vi "MultRRTPlan.vi"(6 "AttackerAvoidArea":bool=TRUE, 7 "Parameters.lvclass":refnum<class "Parameters.lvclass">, 8 "Volta ao redor\nda área?":bool, 9 "Line?":bool, 10 "IA State":T11={"our_robots"=[], "enemy_robots"=[], "balls"=[], "geometry"={"line_width"=0, "field_length"=0, "field_width"=0, "boundary_width"=0, "referee_width"=0, "goal_width"=0, "goal_depth"=0, "goal_wall_width"=0, "center_circle_radius"=0, "defense_radius"=0, "defense_stretch"=0, "free_kick_from_defense_dist"=0, "penalty_spot_from_field_line_dist"=0, "penalty_line_from_spot_dist"=0}, "IA Judge"={"stage"="", "command"="", "our_goalie_id"=0.0, "enemy_goalie_id"=0.0, "command enum"=enum."Halt", "Time"=enum."Azul", "Point"={"x"=0.0, "y"=0.0}}, "Received Timestamp"=timestamp(0 s since 1904-01-01), "Events"={"Touch"=FALSE, "Ball out"=FALSE, "id touch"=0.0, "Ball out of \nVision"=FALSE, "Ball inside \nGoalie area"=FALSE, "Robot not responding"=FALSE, "Robots responding status"=[1.0, 1.0, 1.0, 1.0, 1.0, 1.0], "Enemy Ball \nPossession"=FALSE, "Pass State"=FALSE, "id end of pass"=0.0, "Kick"=FALSE, "Id ini Possession"=0.0, "Ball Possesion"=FALSE, "Id Possesion"=0.0, "Direct Kick"=FALSE, "2nd Strk Ativo"=FALSE}}, 11 "Robot":T1={"id"=0, "function"=enum."Attacker", "x"=0.0, "y"=0.0, "orientation"=0.0, "v_tangent"=0.0, "v_normal"=0.0, "v_ang"=0.0, "kick_x"=0.0, "kick_z"=0.0, "dribble"=FALSE, "Timestamp"=timestamp(0 s since 1904-01-01), "estimatives"={"est_v_tangent"=0.0, "est_v_normal"=0.0, "est_vx"=0.0, "est_vy"=0.0, "Pos Robot Est"=[], "est_v_ang"=0.0}, "dest_x_kick"=0.0, "dest_y_kick"=0.0, "Gap Coord"=[], "States"=enum."GoToTangent", "Path "=[], "Path  Smooth"=[], "Dest"=[], "vx_desired"=0.0, "vy_desired"=0.0, "slowBehavior"=FALSE, "VSSStates"=enum."Pass", "robotKickState"=enum."none", "role"=enum."DefenderArea", "x_k|k"=[]}) -> (2 "Robot Out":T1={"id"=0, "function"=enum."Attacker", "x"=0.0, "y"=0.0, "orientation"=0.0, "v_tangent"=0.0, "v_normal"=0.0, "v_ang"=0.0, "kick_x"=0.0, "kick_z"=0.0, "dribble"=FALSE, "Timestamp"=timestamp(0 s since 1904-01-01), "estimatives"={"est_v_tangent"=0.0, "est_v_normal"=0.0, "est_vx"=0.0, "est_vy"=0.0, "Pos Robot Est"=[], "est_v_ang"=0.0}, "dest_x_kick"=0.0, "dest_y_kick"=0.0, "Gap Coord"=[], "States"=enum."GoToTangent", "Path "=[], "Path  Smooth"=[], "Dest"=[], "vx_desired"=0.0, "vy_desired"=0.0, "slowBehavior"=FALSE, "VSSStates"=enum."Pass", "robotKickState"=enum."none", "role"=enum."DefenderArea", "x_k|k"=[]})   [LabVIEW 2021]
uses:
  Vision_class/Old vision/Controls/AI Robot.ctl
  Vision_class/Old vision/Controls/Functions Enum.ctl
  Controls/estimatives.ctl
  Vision_class/Old vision/Controls/AttackerStates.ctl
  Vision_class/Old vision/Controls/PathDests.ctl
  Vision_class/Old vision/Controls/PathDest.ctl
  Navigation/VSSNavigation/VSSAttackerStates.ctl
  Robot_class/robotKickToStates.ctl
  Robot_class/roles.ctl
  <vilib>/Analysis/Matrix/Datatypes/RealMatrix.ctl
  Vision_class/Old vision/SSL Detection Frame Simple Estimator Cameras VelCmd Folder/Core/AI Input.ctl
  Vision_class/Old vision/SSL Detection Frame Simple Estimator Cameras VelCmd Folder/Core/AI Ball.ctl
  Vision_class/Old vision/SSL Detection Frame Simple Estimator Cameras VelCmd Folder/Core/Field Size.ctl
  Vision_class/Old vision/SSL Detection Frame Simple Estimator Cameras VelCmd Folder/Core/AI Judge.ctl
  Communication_class/Paths/MessageAI_State Folder/Intel/Command Enum.ctl
  Vision_class/Old vision/SSL Detection Frame Simple Estimator Cameras VelCmd Folder/Util/Events/Events.ctl
  Parameters_class/Parameters.lvclass
  Utilities_class/Utilities.lvclass
  <vilib>/Analysis/Matrix/NI_Matrix.lvlib
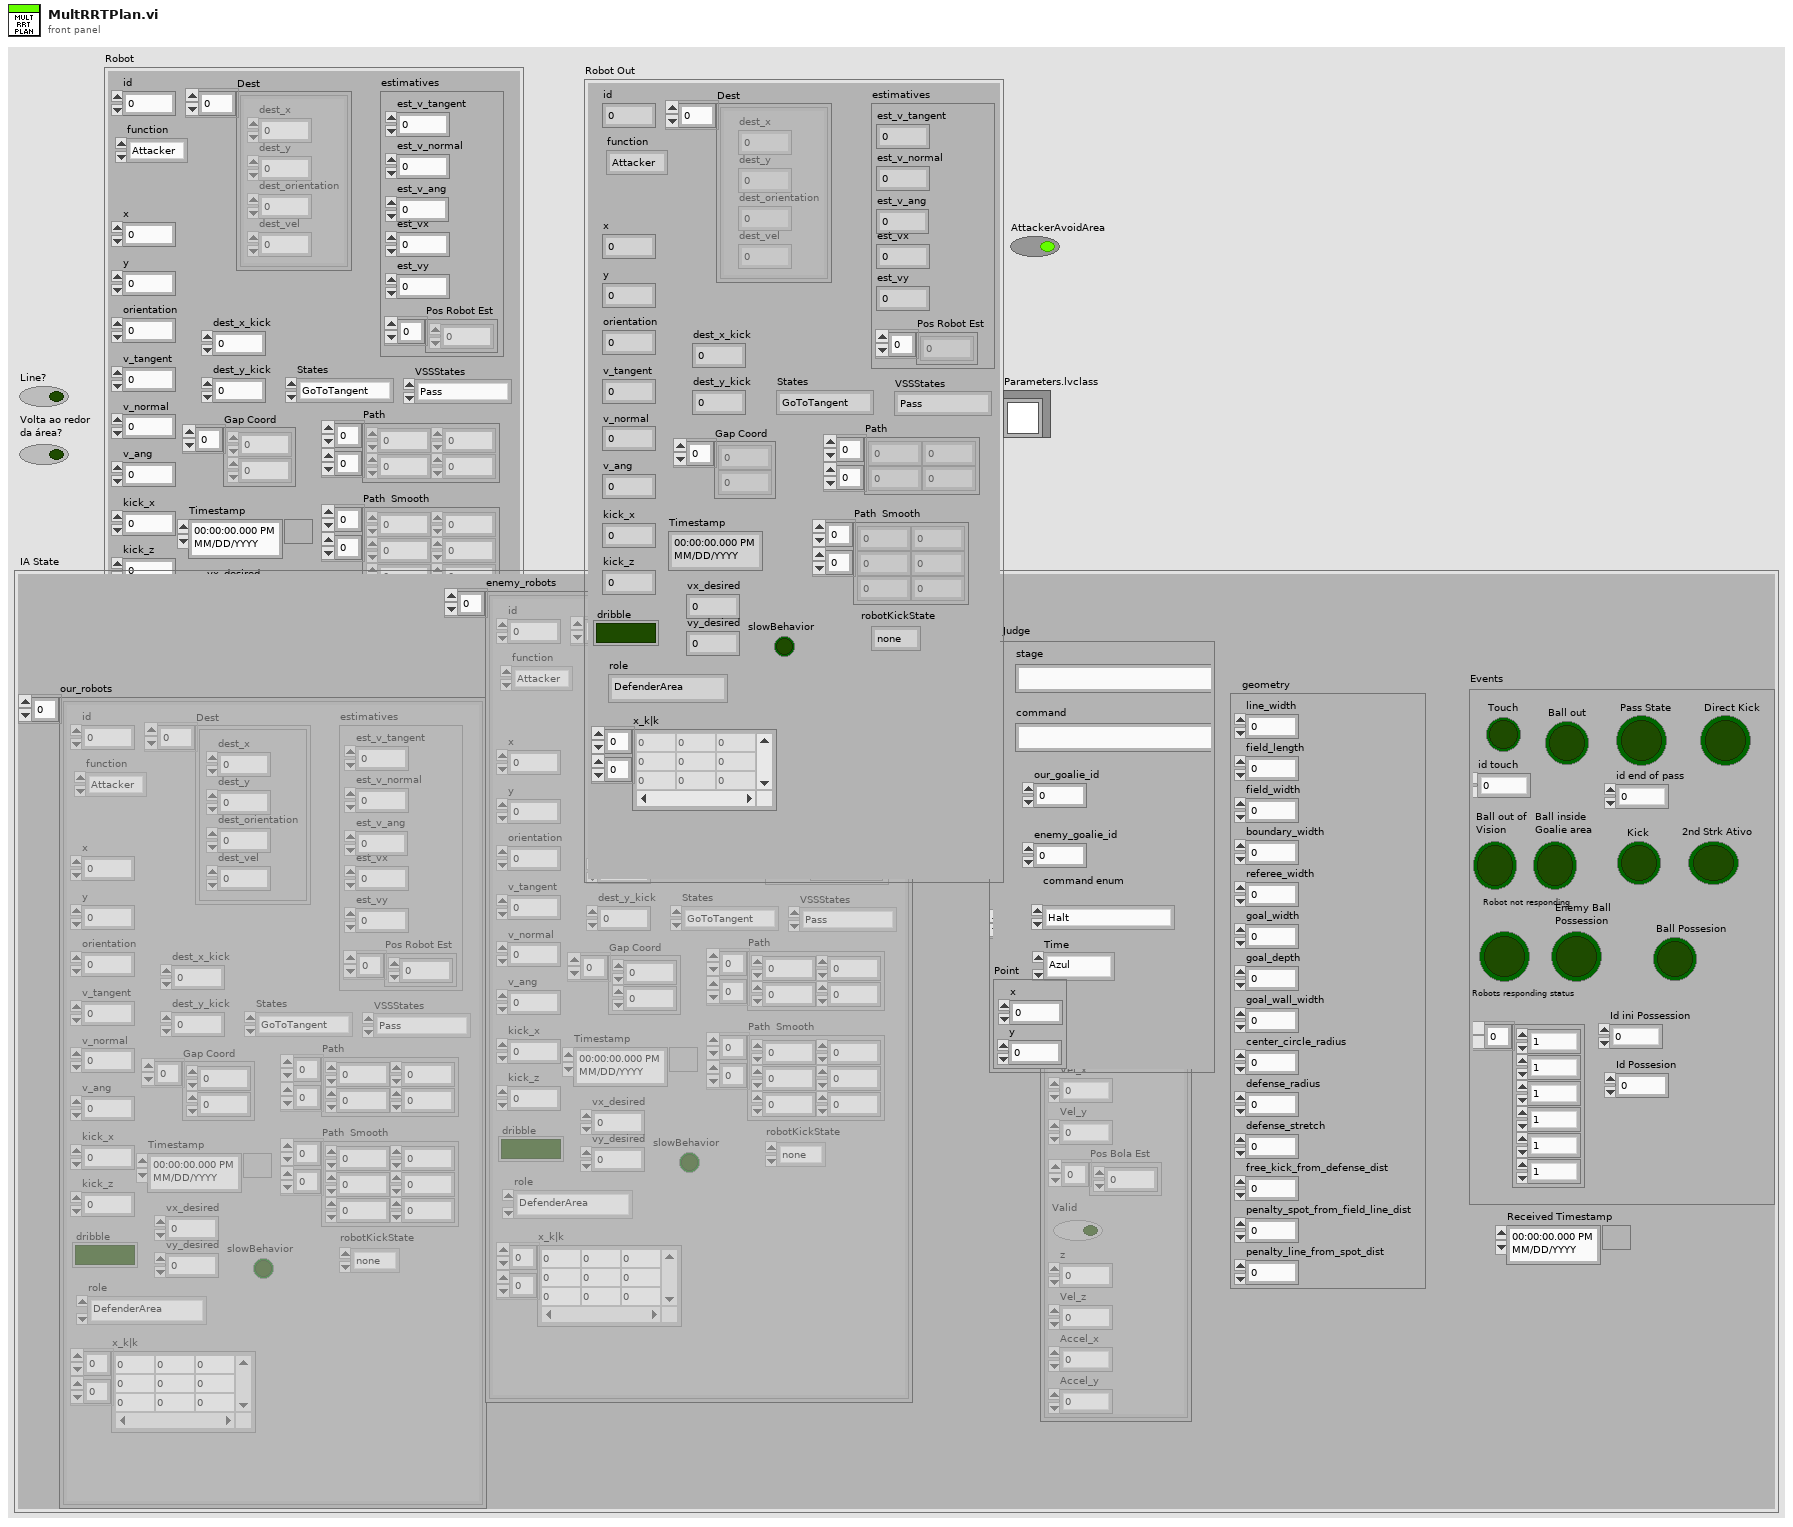
[diagram p1: front panel]
types:
  T1 = typedef "AI Robot.ctl" = cluster{"id":u32, "function":T2, "x":dbl, "y":dbl, "orientation":dbl, "v_tangent":dbl, "v_normal":dbl, "v_ang":dbl, "kick_x":dbl, "kick_z":dbl, "dribble":bool, "Timestamp":timestamp, "estimatives":T3, "dest_x_kick":dbl, "dest_y_kick":dbl, "Gap Coord":dbl[], "States":T4, "Path ":dbl[][], "Path  Smooth":dbl[][], "Dest":T5, "vx_desired":dbl, "vy_desired":dbl, "slowBehavior":bool, "VSSStates":T7, "robotKickState":T8, "role":T9, "x_k|k":T10}
  T2 = typedef "Functions Enum.ctl" = enum16{"2nd Striker", "Attacker", "Goalie", "Defender", "Striker", "Goto 0", "Dummy", "Kicker", "ZigZag 0", "ZigZag 1", "ZigZag 2", "ZigZag 3", "ZigZag 4", "ZigZag 5", "ZigZag 6", "ZigZag 7", "ZigZag 8", ""}
  T3 = typedef "estimatives.ctl" = cluster{"est_v_tangent":dbl, "est_v_normal":dbl, "est_vx":dbl, "est_vy":dbl, "Pos Robot Est":dbl[], "est_v_ang":dbl}
  T4 = typedef "AttackerStates.ctl" = enum16{"Pass", "GoToTangent", "BallGetting", "GoToKick", ""}
  T5 = typedef "PathDests.ctl" = T6[]
  T6 = typedef "PathDest.ctl" = cluster{"dest_x":dbl, "dest_y":dbl, "dest_orientation":dbl, "dest_vel":dbl}
  T7 = typedef "VSSAttackerStates.ctl" = enum16{"Pass", "GoToTangent", "BallGetting", "GoToKick", "Rotate anti-clockwise", "Rotate Clockwise", ""}
  T8 = typedef "robotKickToStates.ctl" = enum16{"shootFromDirect", "avoidCollideBall", "goToBackBall", "none", "walk", "turn", "oldKickToShoot", "oldKickToGoToBackBall", "shoot"}
  T9 = typedef "roles.ctl" = enum16{"SimpleBallPlacement", "BallPlacementAllyPasser", "BallPlacementAllyReceiver", "BallPlacementEnemy", "5Robots5th", "PassBestReceiver", "5Robots4th", "5Robots3rd", "5Robots2nd", "5Robots1st", "PassBestRobot", "WaitPass", "ABCThirdKicker", "ABCFirstKicker", "ABCSecondKicker", "Tabler", "TableFinalizer", "PrepareRollToPassRoller", "PrepareRollToPassReceiver", "SimplePassRoll", "SimplePassRollReceiver", "PenaltyDefense", "PreparePassReceiver 2", "PreparePassReceiver 1", "PassObserver", "Timeout", "Goto", "ZigZag", "None", "BallOutOfField", "DefenderArea", "Duelist", "AttackerStop", "FollowAttacker", "KeeperRole", "KickPenalty", "AttackerAimGoal", "AttackerBlock", "Marker", "Halt", "Shoot", "PassKicker", "PassReceiver", "TestRole", "PenaltyAttacker"}
  T10 = typedef "NI_Matrix.lvlib/RealMatrix.ctl" = dbl[][]
  T11 = typedef "AI Input.ctl" = cluster{"our_robots":T1[], "enemy_robots":T1[], "balls":T12[], "geometry":T13, "IA Judge":T14, "Received Timestamp":timestamp, "Events":T16}
  T12 = typedef "AI Ball.ctl" = cluster{"x":dbl, "y":dbl, "timestamp":timestamp, "Vel_x":dbl, "Vel_y":dbl, "Pos Bola Est":dbl[], "Valid":bool, "z":dbl, "Vel_z":dbl, "Accel_x":dbl, "Accel_y":dbl}
  T13 = typedef "Field Size.ctl" = cluster{"line_width":u32, "field_length":u32, "field_width":u32, "boundary_width":u32, "referee_width":u32, "goal_width":u32, "goal_depth":u32, "goal_wall_width":u32, "center_circle_radius":u32, "defense_radius":u32, "defense_stretch":u32, "free_kick_from_defense_dist":u32, "penalty_spot_from_field_line_dist":u32, "penalty_line_from_spot_dist":u32}
  T14 = typedef "AI Judge.ctl" = cluster{"stage":string, "command":string, "our_goalie_id":dbl, "enemy_goalie_id":dbl, "command enum":T15, "Time":enum16{"Azul", "Amarelo"}, "Point":cluster{"x":sgl, "y":sgl}}
  T15 = typedef "Command Enum.ctl" = enum16{"Halt", "Stop", "Force Start", "PKA Normal Start", "Prepare Kickoff Ally", "PKE Normal Start", "Prepare Kickoff Enemy", "Prepare Penalty Ally", "PPA Normal Start", "Prepare Penalty Enemy", "PPE Normal Start", "Direct Free Enemy", "Direct Free Ally", "Indirect Free Enemy", "Indirect Free Ally", "Timeout Enemy", "Timeout Ally", "Goal Enemy", "Goal Ally", "Ball Placement Enemy", "Ball Placement Ally", "Normal Half Time", "Extra Time Break", "Extra Half Time", "None", "Post Game"}
  T16 = typedef "Events.ctl" = cluster{"Touch":bool, "Ball out":bool, "id touch":dbl, "Ball out of \nVision":bool, "Ball inside \nGoalie area":bool, "Robot not responding":bool, "Robots responding status":dbl[], "Enemy Ball \nPossession":bool, "Pass State":bool, "id end of pass":dbl, "Kick":bool, "Id ini Possession":dbl, "Ball Possesion":bool, "Id Possesion":dbl, "Direct Kick":bool, "2nd Strk Ativo":bool}
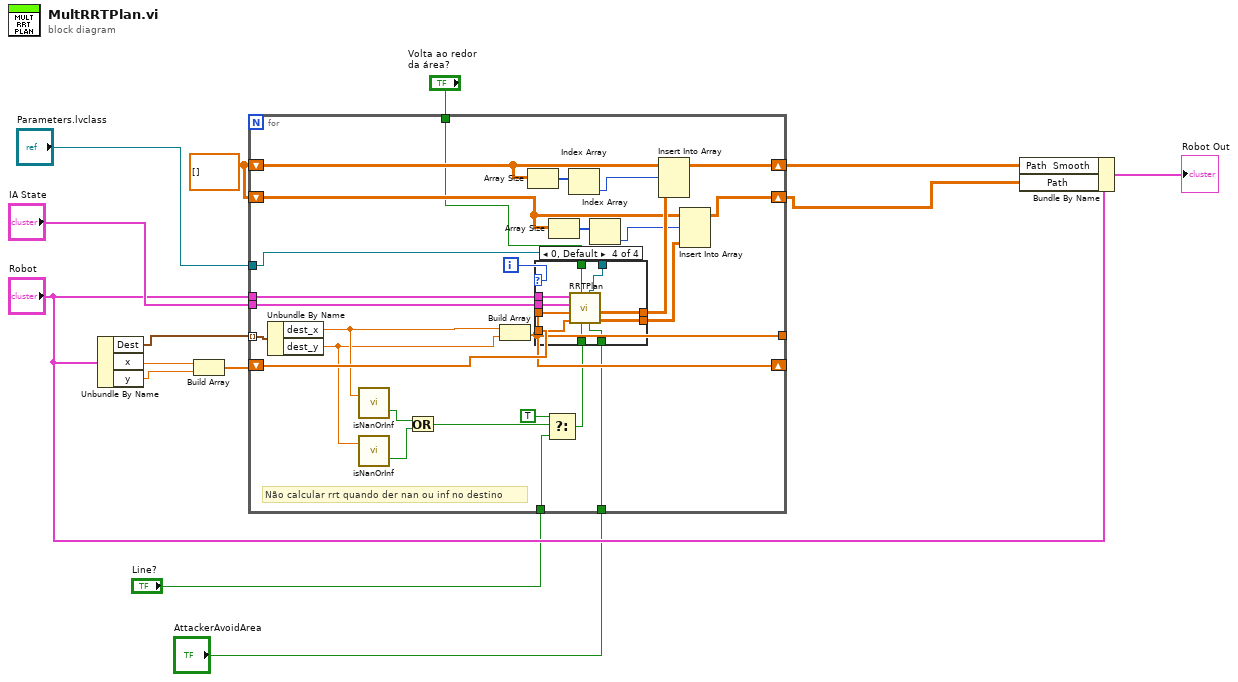
[diagram p0: block diagram]
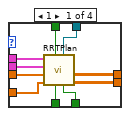
[diagram p2: hidden frame]
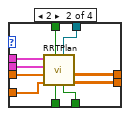
[diagram p3: hidden frame]
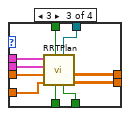
[diagram p4: hidden frame]
diagram:
  w9 = dbl[][] [] ("Path")
  n1 = Unbundle By Name("Robot") -> ("Dest"=w7:T5, "x"=w14:dbl, "y"=w13:dbl)
  n2 = Build Array(w14, w13) -> (w10:dbl[])
  n3 = for {
    tunnel: "Robot" -> [w40]
    tunnel: "IA State" -> [w41]
    shift-right: [w36] -> w5
    shift-left: w9 -> [w35]
    tunnel: w7 -> [w39] mode=indexing
    shift-right: [w32] -> _
    shift-left: w10 -> [w38]
    tunnel: [w32] -> _
    shift-right: [w28] -> w6
    shift-left: w9 -> [w29]
    tunnel: "Line?" -> [w17]
    tunnel: "Volta ao redor\nda área?" -> [w25]
    tunnel: "Parameters.lvclass" -> [w24]
    tunnel: "AttackerAvoidArea" -> [w23]
    i -> [w26]
    # "Não calcular rrt quando der nan ou inf no destino"
    n4 = Unbundle By Name(w39) -> ("dest_x"=w22:dbl, "dest_y"=w21:dbl)
    n5 = call "isNanOrInf.vi"("value"=w22) -> ("narOrInf?"=w20:bool)  [unwired: 13 in, 5 out]
    n6 = call "isNanOrInf.vi"("value"=w21) -> ("narOrInf?"=w19:bool)  [unwired: 13 in, 5 out]
    n7 = Or(x=w20, y=w19) -> (x .or. y?=w18:bool)
    n8 = Build Array(w22, w21) -> (w32:dbl[])
    n9 = Array Size(array=w35) -> (size(s)=w34:i32[])
    n10 = Select(t=TRUE, s=w18, f=w17) -> (s? t:f=w15:bool)
    n11 = case shown="0, Default" w26 {
      tunnel: w41 -> [w51 w61 w71 w81]
      tunnel: w40 -> [w50 w60 w70 w80]
      tunnel: w38 -> [w49 w59 w69 w79]
      tunnel: [w48 w58 w68 w78] -> w37
      tunnel: w32 -> [w47 w57 w67 w77]
      tunnel: [w46 w56 w66 w76] -> w27
      tunnel: w15 -> [w45 w55 w65 w75]
      tunnel: w25 -> [w44 w54 w64 w74]
      tunnel: w24 -> [w43 w53 w63 w73]
      tunnel: w23 -> [w42 w52 w62 w72]
      frame 1 {
        n12 = call "RRTPlan.vi"("AttackerAvoidArea"=w42, "Parameters.lvclass"=w43, "Line?"=w45, "Volta ao redor\nda área?"=w44, "Initial Pos x,y"=w49, "Dest x,y"=w47, "IA State"=w51, "Robot"=w50) -> ("Path"=w46:dbl[][], "Smooth Path"=w48:dbl[][])  [unwired: 2 in]
      }
      frame 2 {
        n13 = call "RRTPlan.vi"("AttackerAvoidArea"=w52, "Parameters.lvclass"=w53, "Line?"=w55, "Volta ao redor\nda área?"=w54, "Initial Pos x,y"=w59, "Dest x,y"=w57, "IA State"=w61, "Robot"=w60) -> ("Path"=w56:dbl[][], "Smooth Path"=w58:dbl[][])  [unwired: 2 in]
      }
      frame 3 {
        n14 = call "RRTPlan.vi"("AttackerAvoidArea"=w62, "Parameters.lvclass"=w63, "Line?"=w65, "Volta ao redor\nda área?"=w64, "Initial Pos x,y"=w69, "Dest x,y"=w67, "IA State"=w71, "Robot"=w70) -> ("Path"=w66:dbl[][], "Smooth Path"=w68:dbl[][])  [unwired: 2 in]
      }
      frame 0, Default {
        n15 = call "RRTPlan.vi"("AttackerAvoidArea"=w72, "Parameters.lvclass"=w73, "Line?"=w75, "Volta ao redor\nda área?"=w74, "Initial Pos x,y"=w79, "Dest x,y"=w77, "IA State"=w81, "Robot"=w80) -> ("Path"=w76:dbl[][], "Smooth Path"=w78:dbl[][])  [unwired: 2 in]
      }
    }
    n16 = Array Size(array=w29) -> (size(s)=w30:i32[])
    n17 = Index Array(array=w34) -> (element=w33:i32)  [unwired: 1 in]
    n18 = Index Array(array=w30) -> (element=w31:i32)  [unwired: 1 in]
    n19 = Insert Into Array(array=w35, index (row)=w33, new element=w37) -> (w36:dbl[][])  [unwired: 1 in]
    n20 = Insert Into Array(array=w29, index (row)=w31, new element=w27) -> (w28:dbl[][])  [unwired: 1 in]
  }
  n21 = Bundle By Name(cluster="Robot", "Path  Smooth"=w5, "Path"=w6) -> (→"Robot Out":T1)
